vi "XML - Get relative RT Driver VI path.vi"(7 "Target Type (Windows)":T1, 8 "error in (no error)":errorcluster, 11 "CD Wizard - Internal Data":T2) -> (0 "error out":errorcluster, 3 "Relative RT Driver VI path":path)   [LabVIEW 2015]
doc: "Create the relative path for the RT Driver VI inside the Configuration LLB based on the name and execution mode of the new custom device."
uses:
  TypDef/CD Wizard - Internal data.ctl
  TypDef/CD Wizard - Execution Mode.ctl
  TypDef/CD Wizard - Extra Page Name and GUID.ctl
  TypDef/Target Type.ctl
  Constants/Constants TypDef/CD Engine lvlib.ctl
  Constants/Constants TypDef/Build Spec Engine.ctl
  Constants/Build Spec Engine.vi
  Constants/CD Engine lvlib.vi
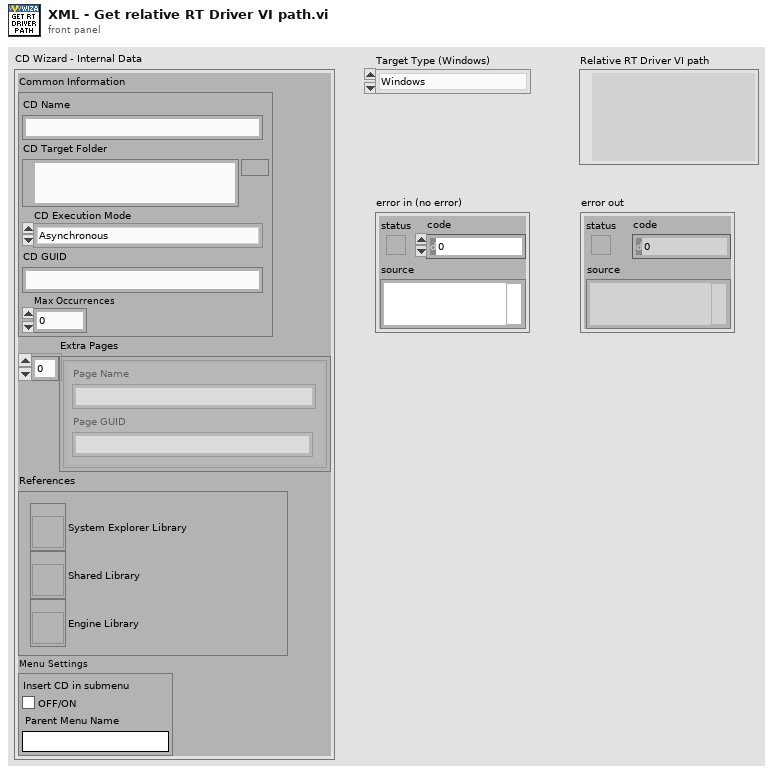
[diagram p1: front panel]
types:
  T1 = typedef "Target Type.ctl" = enum16{"Windows", "VxWorks", "Pharlap", "Linux 32 ARM", "Linux x64"}
  T2 = typedef "CD Wizard - Internal data.ctl" = cluster{"Common Information":cluster{"CD Name":string, "CD Target Folder":path, "CD Execution Mode":T3, "CD GUID":string, "Max Occurrences":u32}, "Extra Pages":T4[], "References":cluster{"System Explorer Library":refnum<vi>, "Shared Library":refnum<vi>, "Engine Library":refnum<vi>}, "Menu Settings":cluster{"Insert CD in submenu":bool, "Parent Menu Name":string}}
  T3 = typedef "CD Wizard - Execution Mode.ctl" = enum16{"Asynchronous", "Inline HW Interface", "Inline Model Interface", "Inline Timing and Sync", "Asynchronous Timing and Sync"}
  T4 = typedef "CD Wizard - Extra Page Name and GUID.ctl" = cluster{"Page Name":string, "Page GUID":string}
  T5 = typedef "CD Engine lvlib.ctl" = enum16{"LibraryFileName", "LibraryFolderName", "Engine.FolderName", "Engine.Init.FolderName", "Engine.Run.FolderName", "Engine.Shutdown.FolderName", "Types.FolderName", "Engine.RT Driver VI.TemplatePath", "Engine.RT Driver VI.FileName"}
  T6 = typedef "Build Spec Engine.ctl" = enum16{"Destinations.LLBWindowsFileName", "Destinations.LLBVxWorksFileName", "Destinations.LLBPharlapFileName", "Destinations.LLBLinuxARMFileName", "Destinations.LLBLinux64FileName"}
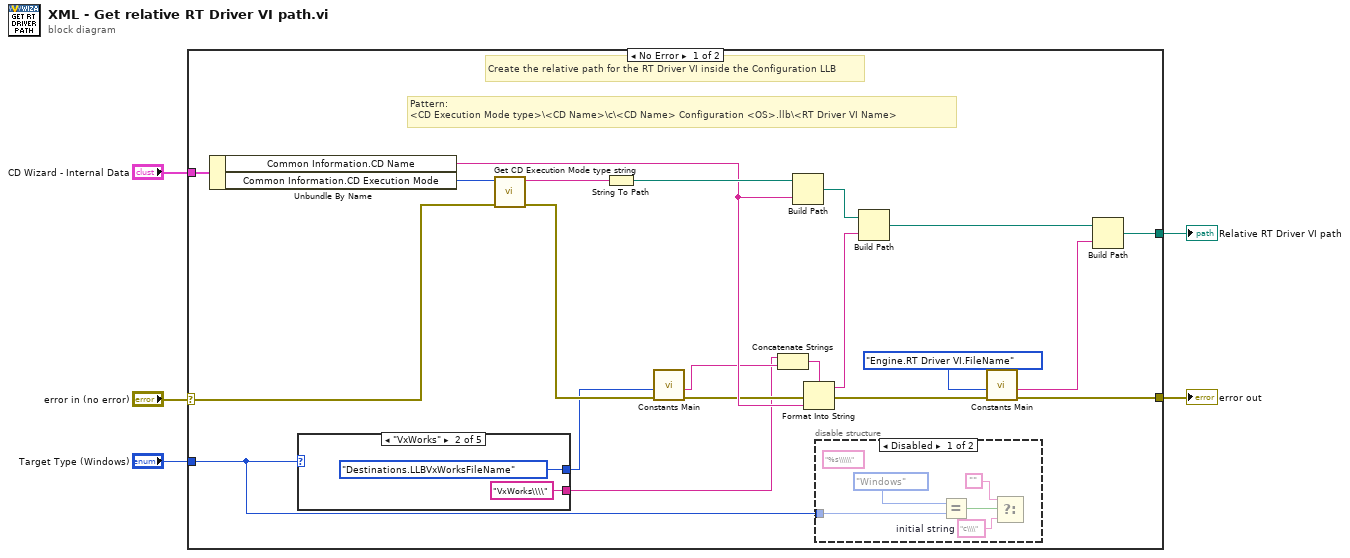
[diagram p0: block diagram]
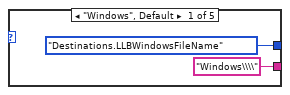
[diagram p3: hidden frame]
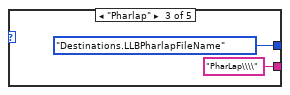
[diagram p4: hidden frame]
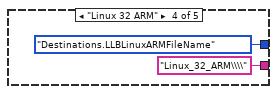
[diagram p5: hidden frame]
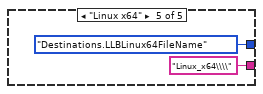
[diagram p6: hidden frame]
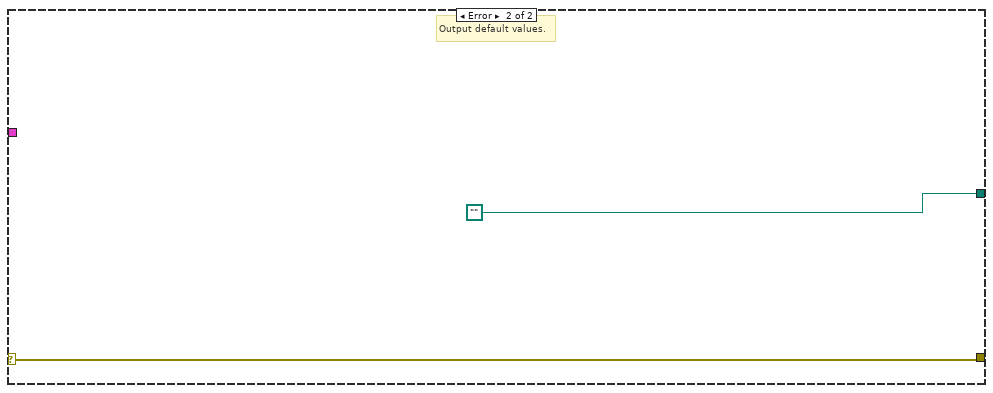
[diagram p7: hidden frame]
diagram:
  n1 = case shown="No Error" "error in (no error)" {
    selector: "error in (no error)" -> [w19 w43]
    tunnel: [w13 w43] -> w2
    tunnel: [w14 path ""] -> w4
    tunnel: "CD Wizard - Internal Data" -> [w24 _]
    tunnel: "Target Type (Windows)" -> [w8 _]
    frame No Error {
      # "Pattern:\n<CD Execution Mode type>\\<CD Name>\\c\\<CD Name> Configuration <OS>.llb\\<RT Driver VI Name>"
      # "Create the relative path for the RT Driver VI inside the Configuration LLB"
      n2 = Unbundle By Name(w24) -> ("Common Information.CD Name"=w22:string, "Common Information.CD Execution Mode"=w20:T3)
      n3 = case shown="\"VxWorks\"" w8 {
        tunnel: [Build_Spec_Engine."Destinations.LLBWindowsFileName" ("Action") Build_Spec_Engine."Destinations.LLBVxWorksFileName" ("Action") Build_Spec_Engine."Destinations.LLBPharlapFileName" ("Action") Build_Spec_Engine."Destinations.LLBLinuxARMFileName" ("Action") Build_Spec_Engine."Destinations.LLBLinux64FileName" ("Action")] -> w11
        tunnel: ["Windows\\\\" ("format string") "VxWorks\\\\" ("format string") "PharLap\\\\" ("format string") "Linux_32_ARM\\\\" ("format string") "Linux_x64\\\\" ("format string")] -> w6
        frame "Windows", Default {
        }
        frame "VxWorks" {
        }
        frame "Pharlap" {
        }
        frame "Linux 32 ARM" {
        }
        frame "Linux x64" {
        }
      }
      n4 = call "Get CD Execution Mode type string.vi"("error in (no error)"=w19, "CD Execution Mode"=w20) -> ("error out"=w18:errorcluster, "Execution Mode type"=w21:string)  [unwired: 8 in]
      n5 = String To Path(string=w21) -> (path=w25:path)
      n6 = call-poly "Constants Main.vi"("error in (no error)"=w18, "Action"=w11) -> ("error out"=w7:errorcluster, "Output"=w10:string)  [unwired: 8 in]
      n7 = Concatenate Strings(w6, w10) -> (w9:string)
      n8 = Build Path(base path=w25, name or relative path=w22) -> (appended path=w23:path)
      n9 = Format Into String(format string=w9, error in=w7, w22) -> (resulting string=w26:string, error out=w16:errorcluster)  [unwired: 1 in]
      n10 = disable-structure shown="Disabled" {
        disable-tunnel: w8 -> [w27 _]
        frame Disabled {
          (unwired) "%s\\\\\\" ("format string")
          w28 = "c\\\\"  # initial string
          n11 = Equal?(x=Target_Type."Windows" ("Target Type (Windows)"), y=w27) -> (x = y?=w30:bool)
          n12 = Select(t="", s=w30, f=w28) -> ()  [unwired: 1 out]
        }
        frame Enabled {
        }
      }
      n13 = Build Path(base path=w23, name or relative path=w26) -> (appended path=w15:path)
      n14 = call-poly "Constants Main.vi"("error in (no error)"=w16, "Action"=CD_Engine_lvlib."Engine.RT Driver VI.FileName") -> ("error out"=w13:errorcluster, "Output"=w12:string)  [unwired: 8 in]
      n15 = Build Path(base path=w15, name or relative path=w12) -> (appended path=w14:path)
    }
    frame Error {
      # "Output default values."
    }
  }
  "error out" <- w2
  "Relative RT Driver VI path" <- w4
